vi "Bundle Actor Core Refs.vi"(8 "error in (no error)":errorcluster, 10 "ControlReferenceConstants":refnum<vi>[](array[refnum]), 11 "VI":refnum<vi>) -> (0 "error out":errorcluster)   [LabVIEW 2020, in "Add to Private Data.lvlib"]
uses:
  Add to Private Data.lvlib
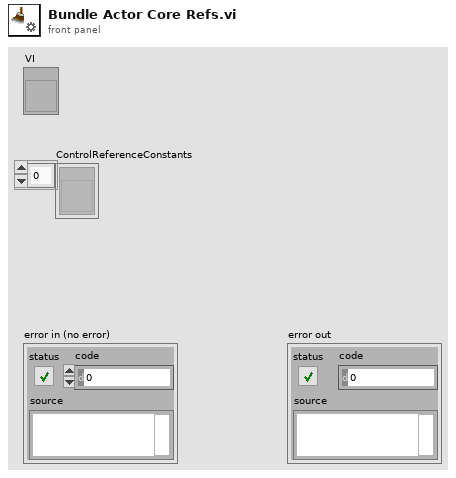
[diagram p1: front panel]
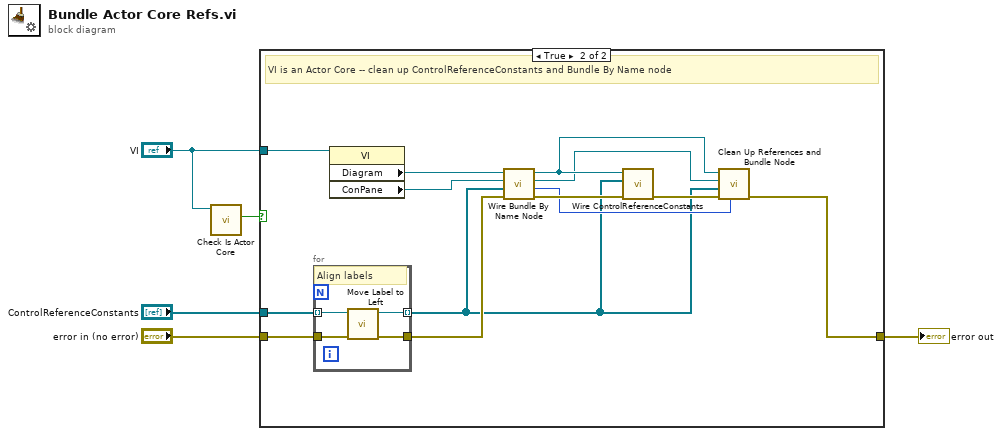
[diagram p0: block diagram]
diagram:
  n1 = call "Check Is Actor Core.vi"("VI in"="VI") -> ("Is Actor Core?"=w2:bool)  [unwired: 9 in, 1 out]
  n2 = case shown="True" w2 {
    tunnel: [w6 w12] -> w5
    tunnel: "error in (no error)" -> [w6 w19]
    tunnel: "ControlReferenceConstants" -> [_ w18]
    tunnel: "VI" -> [_ w17]
    frame False {
      # "For now, do nothing to non-Actors"
    }
    frame True {
      # "VI is an Actor Core -- clean up ControlReferenceConstants and Bundle By Name node"
      n3 = for {
        tunnel: w18 -> [w22] mode=indexing
        tunnel: w19 -> [w21]
        tunnel: [w23] -> w15
        tunnel: [w20] -> w7 mode=indexing
        # "Align labels"
        n4 = call "Move Label to Left.vi"("error in (no error)"=w21, "ControlReferenceConstant in"=w22) -> ("error out"=w23:errorcluster, "ControlReferenceConstant out"=w20:refnum<vi>)  [unwired: 8 in]
      }
      n5 = property class="VI"(reference=w17) -> ("Diagram"=w16:refnum<vi>, "ConPane"=w8:refnum<vi>)  [unwired: 1 in, 2 out]
      n6 = call "Wire Bundle By Name Node.vi"("error in (no error)"=w15, "ControlReferenceConstants"=w7, "ConPane"=w8, "TopLevelDiagram in"=w16) -> ("error out"=w14:errorcluster, "Total Number of Inputs"=w9:i32, "Actor Input ControlTerminal"=w10:refnum<vi>, "NamedBundler"=w11:refnum<vi>)  [unwired: 4 in]
      n7 = call "Wire ControlReferenceConstants.vi"("error in (no error)"=w14, "ControlReferenceConstants"=w7, "NamedBundler"=w11) -> ("error out"=w13:errorcluster)  [unwired: 6 in, 2 out]
      n8 = call "Clean Up References and Bundle Node.vi"("Total Number of Inputs"=w9, "error in (no error)"=w13, "ControlReferenceConstants"=w7, "Actor Input ControlTerminal"=w10, "NamedBundler"=w11) -> ("error out"=w12:errorcluster)  [unwired: 6 in]
    }
  }
  "error out" <- w5
